vi "Main_with_simulator.vi"() -> ()   [LabVIEW 2013]
doc: "Main code that will run on the robot and contains all the logic and hardware interfaces."
uses:
  Data/TypeDefs/UTM Location.ctl
  Data/TypeDefs/Sail Set Suggestions.ctl
  Data/TypeDefs/Rudder Set Suggestions.ctl
  Data/TypeDefs/OverrideInformation.ctl
  Data/TypeDefs/OverrideMode.ctl
  Logic/Classes/Missions/GenericMission/GenericMission.lvclass
  Logic/Classes/Obstacle/Obstacle.lvclass
  Data/TypeDefs/BoatType.ctl
  Logic/Classes/Logger/Logger.lvclass
panel:
  in  "Boat Type":T1=enum."Damn Yankee"
  in  "Do Basic Logging? (T)":bool
  out "Logging file path":path
  out "Missions":refnum<class "GenericMission.lvclass">[](array[class])
  out "Obstacles":refnum<class "Obstacle.lvclass">[](array[class])
  out "Finished Missions":refnum<class "GenericMission.lvclass">[](array[class])
  out "OverrideInformation":T2={"OverrideMode"=enum."Rudder", "SailSetting"={"MainSailSuggestion"=0.0, "JibSailSuggestion"=0.0}, "Rudder Setpoint"=0.0, "Sim_Wind_Speed"=0.0, "Sim_Wind_Heading"=0.0} {"SailSetting"."MainSailSuggestion" min=0.0 max=1.0; "SailSetting"."JibSailSuggestion" min=0.0 max=1.0; "Rudder Setpoint" min=-0.95 max=0.95 scale=1.0..-1.0}
  out "DisplayCounter":i32
  out "AbsWindDirection":dbl
  out "IronsRange":dbl
  out "RudderPosition":T5 min=-0.95 max=0.95 scale=1.0..-1.0
  out "SailPositions":T4 {"MainSailSuggestion" min=0.0 max=1.0; "JibSailSuggestion" min=0.0 max=1.0}
  out "RelWindDirection":dbl
  out "RateOfTurn":dbl
  out "BoatLocation":T6 {"North" format="%#_10f"; "East" format="%#_8f"}
  out "BoatDirection":dbl
  out "WindSpeed":dbl
  out "BoatSpeed":dbl
  in  "XBee Serial Port":refnum<visa-resource-name>="COM8"
  in  "stop":bool
  # "ALL THE DEBUG INFO - Eric"
  # "SET THIS BEFORE RUNNING\nOR YOU WILL NEED TO\nRESTART THE CODE!!!"
  # "For Little Boat Initialization"
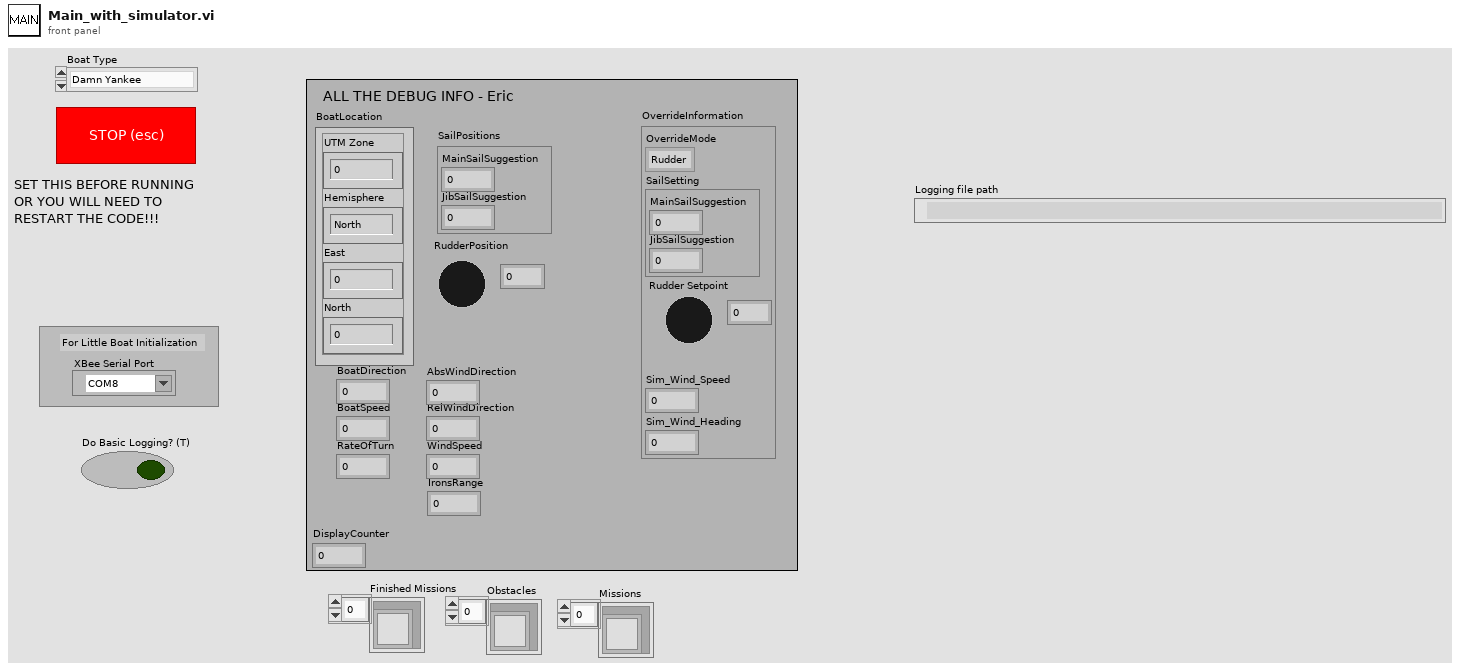
[diagram p1: front panel]
types:
  T1 = typedef "BoatType.ctl" = enum16{"Blackbody Radiation", "Simulator", "ReadLog", "Little boats", "Damn Yankee"}
  T2 = typedef "OverrideInformation.ctl" = cluster{"OverrideMode":T3, "SailSetting":T4, "Rudder Setpoint":T5, "Sim_Wind_Speed":dbl, "Sim_Wind_Heading":dbl}
  T3 = typedef "OverrideMode.ctl" = enum16{"None", "Rudder", "Sails", "Both"}
  T4 = typedef "Sail Set Suggestions.ctl" = cluster{"MainSailSuggestion":dbl, "JibSailSuggestion":dbl}
  T5 = typedef "Rudder Set Suggestions.ctl" = dbl
  T6 = typedef "UTM Location.ctl" = cluster{"UTM Zone":dbl, "Hemisphere":enum16{"North", "South"}, "East":dbl, "North":dbl}
  T7 = typedef "MissionNotifiers.ctl" = cluster{"Missions":refnum<notifier>, "Finished Missions":refnum<notifier>, "Obstacles":refnum<notifier>}
  T8 = typedef "Notifiers.ctl" = cluster{"BoatSpeed":refnum<notifier>, "WindSpeed":refnum<notifier>, "EStop":refnum<notifier>, "BoatDirection":refnum<notifier>, "Luffing":refnum<notifier>, "RudderForce":refnum<notifier>, "BatteryVoltage":refnum<notifier>, "StayForces":refnum<notifier>, "BoatLocation":refnum<notifier>, "Pitch":refnum<notifier>, "Roll":refnum<notifier>, "RateOfTurn":refnum<notifier>, "RelWindDirection":refnum<notifier>, "SailPositions":refnum<notifier>, "RudderPosition":refnum<notifier>, "IronsRange":refnum<notifier>, "AbsWindDirection":refnum<notifier>, "OverrideInformation":refnum<notifier>, "DynamixelTorques":refnum<notifier>, "MotorSetup":refnum<notifier>, "AirmarStatus":refnum<notifier>, "HardwareOnline?":refnum<notifier>, "Sim_ActualSailPositions [0,1]":refnum<notifier>, "DynamixelCycleTracker":refnum<notifier>, "BoatVelocityDirection":refnum<notifier>, "SimWindHeading(rad)":refnum<notifier>, "SimWindSpeed(m/s)":refnum<notifier>, "RCInputValues":refnum<notifier>, "Finished Waypoints":refnum<notifier>, "DesiredHeading":refnum<notifier>, "Latest Mission ID":refnum<notifier>, "Latest Obstacle ID":refnum<notifier>, "DownwindDiscouragedRange":refnum<notifier>, "Tack Range":refnum<notifier>, "Tacking?":refnum<notifier>}
  T9 = typedef "Queues.ctl" = cluster{"Waypoints":refnum<queue>}
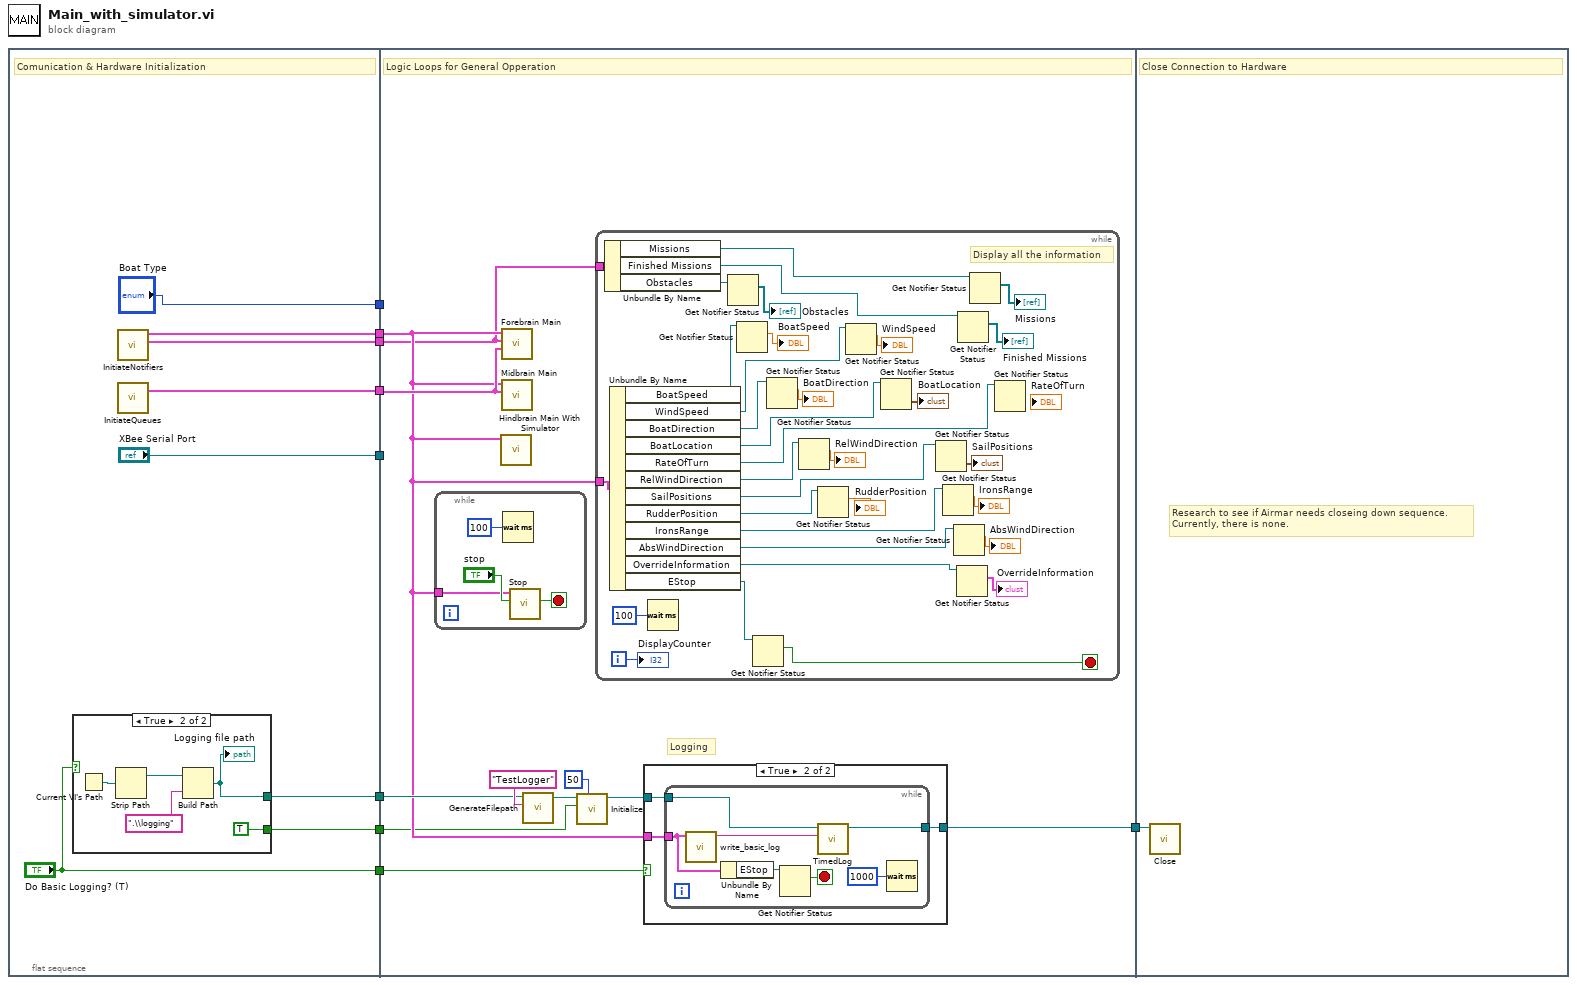
[diagram p0: block diagram]
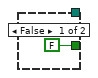
[diagram p2: hidden frame]
diagram:
  n1 = flat-sequence {
    tunnel: [w17] -> w9
    tunnel: ["Boat Type"] -> w8
    tunnel: [w16] -> w7
    tunnel: ["XBee Serial Port"] -> w6
    tunnel: [w14] -> w5
    tunnel: [w13] -> w3
    tunnel: [w12] -> w2
    tunnel: ["Do Basic Logging? (T)"] -> w1
    tunnel: w9 -> [w34]
    tunnel: w8 -> [_]
    tunnel: w7 -> [w27]
    tunnel: w6 -> [_]
    tunnel: w5 -> [w26]
    tunnel: [w30] -> w4
    tunnel: w3 -> [w28]
    tunnel: w2 -> [w25]
    tunnel: w1 -> [w24]
    tunnel: w4 -> [w83]
    frame #0 {
      # "Comunication & Hardware Initialization"
      n2 = case shown="True" "Do Basic Logging? (T)" {
        tunnel: [_ w22] -> w13
        tunnel: [FALSE ("Enable? (T)") TRUE ("Enable? (T)")] -> w12
        frame False {
        }
        frame True {
          n3 = Current VI's Path() -> (path=w20:path)
          n4 = Strip Path(path=w20) -> (stripped path=w19:path)  [unwired: 1 out]
          n5 = Build Path(base path=w19, name or relative path=".\\logging") -> (appended path=w22:path)
          "Logging file path" <- w22
        }
      }
      n6 = call "InitiateNotifiers.vi"() -> ("Mission Notifiers"=w14:T7, "NotifierReferences"=w16:T8)  [unwired: 9 in, 1 out]
      n7 = call "InitiateQueues.vi"() -> ("Queue References"=w17:T9)  [unwired: 3 in]
    }
    frame #1 {
      # "Logging"
      # "Logic Loops for General Opperation"
      n8 = while {
        tunnel: w27 -> [w79]
        stop <- w80 stop-if-true
        n9 = Wait (ms)(milliseconds to wait=u32 100) -> ()  [unwired: 1 out]
        n10 = call "Stop.vi"("StopButton"="stop", "NotifierReff"=w79) -> ("StopOut"=w80:bool)  [unwired: 9 in]
      }
      n11 = call "Hindbrain Main With Simulator.vi"("NotifierReff"=w27) -> ()  [unwired: 11 in]
      n12 = call "Forebrain Main.vi"("QueueRef"=w34, "Mission Notifiers"=w26, "NotifierReff"=w27) -> ()  [unwired: 8 in, 1 out]
      n13 = call "Midbrain Main.vi"("Waypoint Queue Ref"=w34, "Notifier Ref"=w27) -> ()  [unwired: 10 in]
      n14 = call "GenerateFilepath.vi"("Identifier"="TestLogger", "Data storage folder"=w28) -> ("File path out"=w31:path)  [unwired: 8 in, 1 out]
      n15 = call "Initialize.vi"("buffer size"=50, "Enable? (T)"=w25, "File path"=w31) -> ("Logger out"=w32:refnum<class "Logger.lvclass">)  [unwired: 7 in, 1 out]
      n16 = while {
        tunnel: w27 -> [w77]
        tunnel: w26 -> [w52]
        i -> [w57]
        stop <- w54 stop-if-true
        # "Display all the information"
        n17 = Unbundle By Name(w52) -> ("Missions"=w47:refnum<notifier>, "Finished Missions"=w49:refnum<notifier>, "Obstacles"=w51:refnum<notifier>)
        n18 = Unbundle By Name(w77) -> ("BoatSpeed"=w76:refnum<notifier>, "WindSpeed"=w74:refnum<notifier>, "BoatDirection"=w71:refnum<notifier>, "BoatLocation"=w70:refnum<notifier>, "RateOfTurn"=w68:refnum<notifier>, "RelWindDirection"=w66:refnum<notifier>, "SailPositions"=w65:refnum<notifier>, "RudderPosition"=w63:refnum<notifier>, "IronsRange"=w60:refnum<notifier>, "AbsWindDirection"=w58:refnum<notifier>, "OverrideInformation"=w56:refnum<notifier>, "EStop"=w53:refnum<notifier>)
        n19 = Wait (ms)(milliseconds to wait=u32 100) -> ()  [unwired: 1 out]
        n20 = Get Notifier Status(notifier=w51) -> (current notification=→"Obstacles":refnum<class "Obstacle.lvclass">[])  [unwired: 1 in, 4 out]
        n21 = Get Notifier Status(notifier=w76) -> (current notification=→"BoatSpeed":dbl)  [unwired: 1 in, 4 out]
        n22 = Get Notifier Status(notifier=w53) -> (current notification=w54:bool)  [unwired: 1 in, 4 out]
        n23 = Get Notifier Status(notifier=w71) -> (current notification=→"BoatDirection":dbl)  [unwired: 1 in, 4 out]
        n24 = Get Notifier Status(notifier=w66) -> (current notification=→"RelWindDirection":dbl)  [unwired: 1 in, 4 out]
        n25 = Get Notifier Status(notifier=w63) -> (current notification=→"RudderPosition":T5)  [unwired: 1 in, 4 out]
        n26 = Get Notifier Status(notifier=w74) -> (current notification=→"WindSpeed":dbl)  [unwired: 1 in, 4 out]
        n27 = Get Notifier Status(notifier=w70) -> (current notification=→"BoatLocation":T6)  [unwired: 1 in, 4 out]
        n28 = Get Notifier Status(notifier=w65) -> (current notification=→"SailPositions":T4)  [unwired: 1 in, 4 out]
        n29 = Get Notifier Status(notifier=w60) -> (current notification=→"IronsRange":dbl)  [unwired: 1 in, 4 out]
        n30 = Get Notifier Status(notifier=w58) -> (current notification=→"AbsWindDirection":dbl)  [unwired: 1 in, 4 out]
        n31 = Get Notifier Status(notifier=w56) -> (current notification=→"OverrideInformation":T2)  [unwired: 1 in, 4 out]
        n32 = Get Notifier Status(notifier=w49) -> (current notification=→"Finished Missions":refnum<class "GenericMission.lvclass">[])  [unwired: 1 in, 4 out]
        n33 = Get Notifier Status(notifier=w47) -> (current notification=→"Missions":refnum<class "GenericMission.lvclass">[])  [unwired: 1 in, 4 out]
        n34 = Get Notifier Status(notifier=w68) -> ()  [unwired: 1 in, 5 out]
        "DisplayCounter" <- w57
      }
      n35 = case shown="True" w24 {
        tunnel: w32 -> [w35 w38]
        tunnel: [w35 w37] -> w30
        tunnel: w27 -> [_ w36]
        frame False {
        }
        frame True {
          n36 = while {
            tunnel: w36 -> [w40]
            tunnel: w38 -> [w42]
            tunnel: [w41] -> w37
            stop <- w44 stop-if-true
            n37 = call "write_basic_log.vi"("NotifierReff"=w40) -> ("xml string"=w39:string)  [unwired: 10 in]
            n38 = Unbundle By Name(w40) -> ("EStop"=w45:refnum<notifier>)
            n39 = Get Notifier Status(notifier=w45) -> (current notification=w44:bool)  [unwired: 1 in, 4 out]
            n40 = call "TimedLog.vi"("Message"=w39, "Logger in"=w42) -> ("Logger out"=w41:refnum<class "Logger.lvclass">)  [unwired: 7 in, 2 out]
            n41 = Wait (ms)(milliseconds to wait=u32 1000) -> ()  [unwired: 1 out]
          }
        }
      }
    }
    frame #2 {
      # "Research to see if Airmar needs closeing down sequence.\nCurrently, there is none."
      # "Close Connection to Hardware"
      n42 = call "Close.vi"("Logger in"=w83) -> ()  [unwired: 10 in, 1 out]
    }
  }
